vi "Execute.vi"(8 "error in (no error)":errorcluster, 10 "Context in":refnum<class "Context.lvclass">, 11 "Test One Test Command in":refnum<class "Test One Test Command.lvclass">) -> (0 "error out":errorcluster, 2 "Context out":refnum<class "Context.lvclass">, 3 "Test One Test Command out":refnum<class "Test One Test Command.lvclass">)   [LabVIEW 2016, in "Test One Test Command.lvclass"]
uses:
  Test One Test Command.lvclass
  Command/Command.lvclass
  Context/Context.lvclass
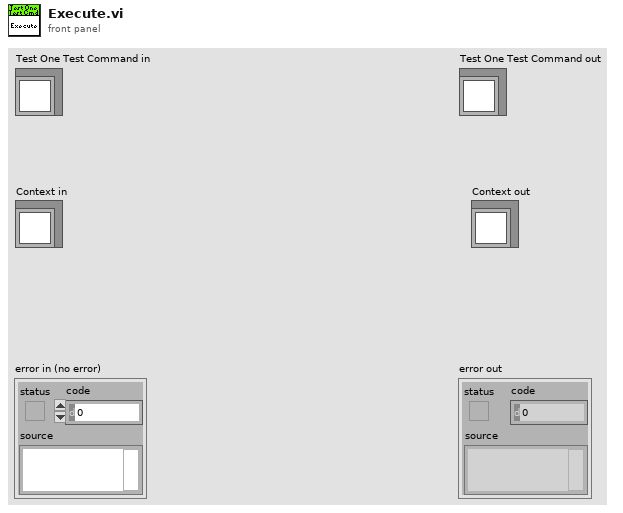
[diagram p1: front panel]
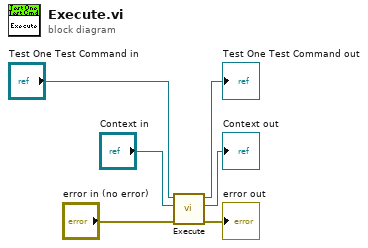
[diagram p0: block diagram]
diagram:
  n1 = call-parent "Execute.vi"("error in (no error)"="error in (no error)", "Context in"="Context in", "Command in"="Test One Test Command in") -> ("error out"=→"error out":errorcluster, "Context out"=→"Context out":refnum<class "Context.lvclass">, "Command out"=→"Test One Test Command out":refnum<class "Test One Test Command.lvclass">)  [unwired: 6 in]
